vi "IX83 Reply Value.vi"(0 "Connection ID":refnum<k5>, 7 "Reply":string, 11 "Error In":errorcluster) -> (4 "Connection ID Out":refnum<k5>, 6 "Reply":string, 8 "Bool":bool, 10 "Value":dbl, 15 "Error Out":errorcluster)   [LabVIEW 2020]
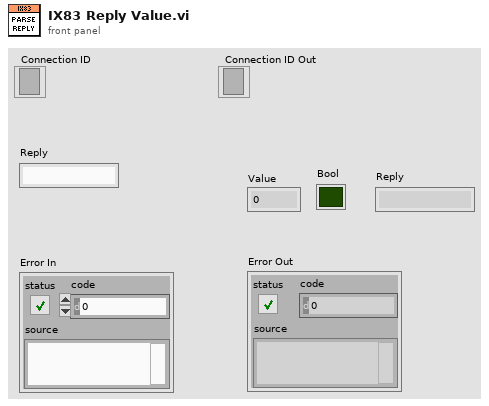
[diagram p1: front panel]
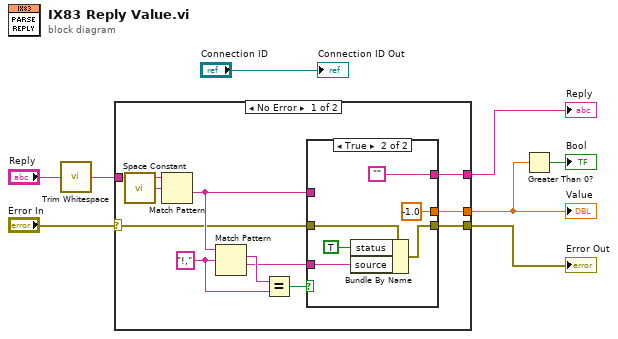
[diagram p0: block diagram]
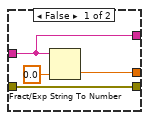
[diagram p2: hidden frame]
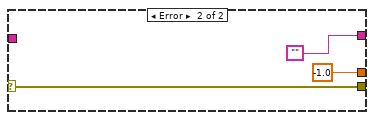
[diagram p3: hidden frame]
diagram:
  n1 = call <vilib>:"Trim Whitespace.vi"("string"="Reply") -> ("trimmed string"=w5:string)  [unwired: 1 in]
  n2 = case shown="No Error" "Error In" {
    selector: "Error In" -> [w13 w31]
    tunnel: w5 -> [w19 _]
    tunnel: [w11 -1.0] -> w3
    tunnel: [w10 w31] -> w2
    tunnel: [w9 ""] -> w1
    frame No Error {
      w16 = "!," ("regular expression")
      n3 = call <vilib>:"Space Constant.vi"() -> ("String"=w18:string)
      n4 = Match Pattern(string=w19, regular expression=w18) -> (after substring=w14:string)  [unwired: 1 in, 3 out]
      n5 = Match Pattern(string=w14, regular expression=w16) -> (match substring=w17:string, after substring=w12:string)  [unwired: 1 in, 2 out]
      n6 = Equal?(x=w17, y=w16) -> (x = y?=w15:bool)
      n7 = case shown="True" w15 {
        tunnel: w14 -> [w20 _]
        tunnel: w13 -> [w21 w29]
        tunnel: w12 -> [_ w27]
        tunnel: [w22 -1.0] -> w11
        tunnel: [w21 w26] -> w10
        tunnel: [w20 ""] -> w9
        frame False {
          n8 = Fract/Exp String To Number(string=w20, default (0 dbl)=0.0 ("default (0 DBL)")) -> (number=w22:dbl)  [unwired: 2 in, 1 out]
        }
        frame True {
          n9 = Bundle By Name(cluster=w29, "status"=TRUE, "source"=w27) -> (w26:errorcluster)
        }
      }
    }
    frame Error {
    }
  }
  "Error Out" <- w2
  "Value" <- w3
  "Reply" <- w1
  n10 = Greater Than 0?(x=w3) -> (x > 0?=→"Bool":bool)
  "Connection ID Out" <- "Connection ID"
